vi "runBECBasic.vi"() -> ()   [LabVIEW 2011, in "run.lvlib"]
doc: "Launch the applications that will control the experiment.\n\n1) Load Database, filesystem, file neologist.\n2) Start a clock for the DDS rf card.\n3) Launch Experiment Runner front viewer\n4) Launch Hardware Controller in the backend."
uses:
  run.lvlib
  Viewers/Editors/ExperimentRunner/ExperimentRunner.lvclass
  HWController/HWController.lvclass
  HWController/BECHWCBasic/BECHWCBasic.lvclass
  HWController/HWControllerEvents/HWControllerEvents.lvclass
  Tools/DatabaseHelpers/DbConnection/DeviceDataBase/deviceDataBase.lvclass
  HWController/HardwareConfiguration/HWConfiguration.lvclass
  Viewers/Editors/ExperimentRunner/RunExperiment/ExperimentControl.lvclass
  Viewers/Editors/ExperimentRunner/Events/ExperimentControlEvents.lvclass
  HWController/AtomChipHWC/AtomChipHWC.lvclass
  Tools/Filing/FileSystem/FileSystem.lvclass
  Tools/Filing/FileNeologist/FileNeologist.lvclass
  Tools/Filing.lvlib
  Tools/DatabaseHelpers.lvlib
  Events/Event.lvclass
  Viewers/ExperimentControl.lvlib
panel:
  in  "Experiment":enum16{"BEC1", "AtomChip"}(ring)=enum."AtomChip"
  in  "Camera on?":bool
  in  "Hardware On?":bool=TRUE
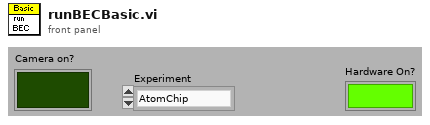
[diagram p1: front panel]
types:
  T1 = enum32{"Invalid", "Standard", "Closed", "Hidden", "Minimized", "Maximized"}
  T2 = enum32{"Bad", "Idle", "Run top level", "Running"}
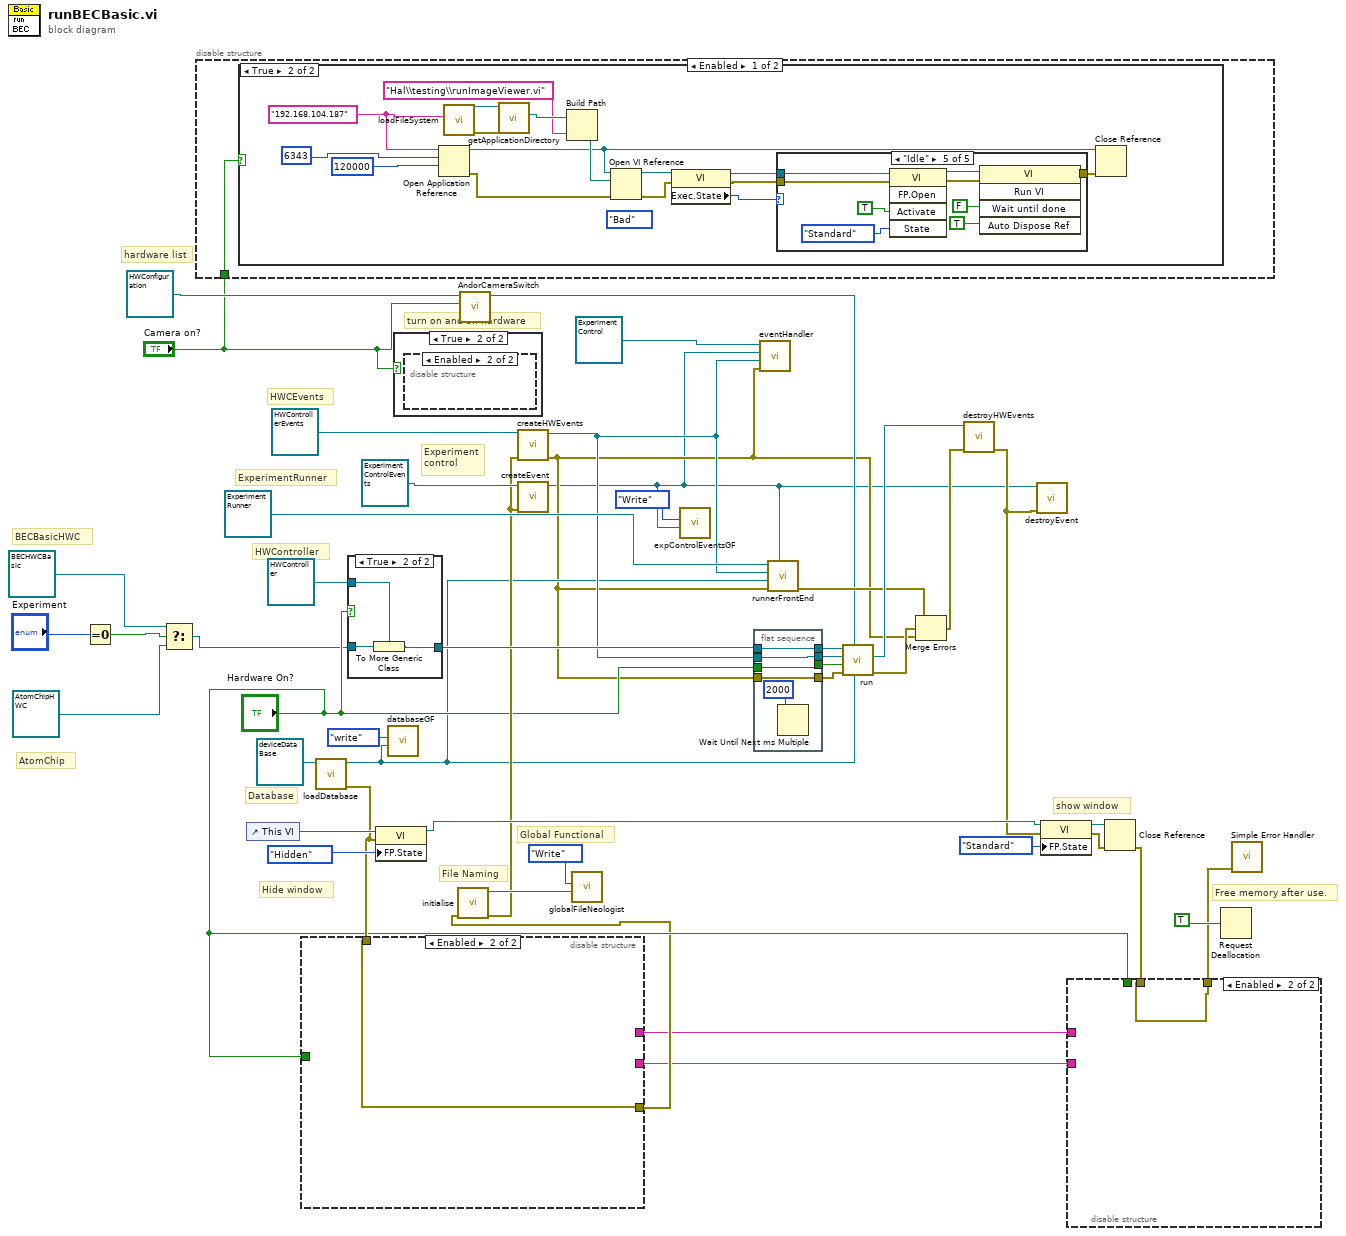
[diagram p0: block diagram]
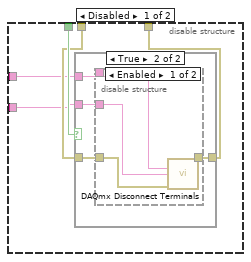
[diagram p8: hidden frame]
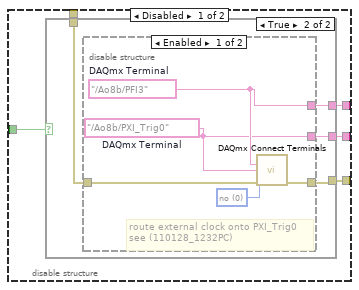
[diagram p11: hidden frame]
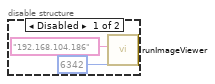
[diagram p15: hidden frame]
diagram:
  # "turn on and off hardware"
  # "AtomChip"
  # "Experiment\ncontrol"
  # "hardware list"
  # "Free memory after use."
  # "BECBasicHWC"
  # "Hide window"
  # "show window"
  # "Database"
  # "File Naming"
  # "Global Functional"
  # "HWController"
  # "ExperimentRunner"
  # "HWCEvents"
  n1 = Equal To 0?(x="Experiment") -> (x = 0?=w7:bool)
  n2 = Select(t=refnum<class "BECHWCBasic.lvclass"> refnum ("Hardware:HWControllers.lvlib:BECHWCBasic.lvclass"), s=w7, f=refnum<class "AtomChipHWC.lvclass"> refnum ("Hardware:HWControllers.lvlib:AtomChipHWC.lvclass")) -> (s? t:f=w4:refnum<class "HWController.lvclass">)
  n3 = disable-structure shown="Enabled" {
    disable-tunnel: "Camera on?" -> [w48 _]
    frame Enabled {
      n4 = case shown="True" w48 {
        frame False {
        }
        frame True {
          (unwired) T2."Bad" ("Execution:State")
          w55 = "192.168.104.187" ("remote address")
          n5 = Open Application Reference(9:120000 ("timeout ms (60000)"), 10:6343, 11:w55) -> (0:w64:errorcluster, 3:w58:refnum<vi>)  [unwired: 1 in]
          n6 = call "loadFileSystem.vi"("computer name"=w55) -> ("error out"=w62:errorcluster, "FileSystem out"=w63:refnum<class "FileSystem.lvclass">)  [unwired: 9 in]
          n7 = call-dynamic "getApplicationDirectory.vi"("error in (no error)"=w62, "FileSystem.lvclass in"=w63) -> ("ApplicationDirectory"=w61:path)  [unwired: 7 in, 2 out]
          n8 = Build Path(base path=w61, name or relative path="Hal\\testing\\runImageViewer.vi") -> (appended path=w59:path)
          n9 = Open VI Reference(application reference (local)=w58, vi path=w59, error in (no error)=w64) -> (vi reference=w53:refnum<vi>, error out=w52:errorcluster)  [unwired: 3 in]
          n10 = property class="VI"(reference=w53, error in=w52) -> (reference out=w50:refnum<vi>, error out=w51:errorcluster, "Exec.State"=w49:T2)
          n11 = case shown="\"Idle\"" w49 {
            tunnel: [w65 w66 w67 w68 w75] -> w57
            tunnel: w51 -> [w65 w66 w67 w68 w70]
            tunnel: w50 -> [_ _ _ _ w69]
            frame "Bad" {
            }
            frame Default {
            }
            frame "Running" {
            }
            frame "Run top level" {
            }
            frame "Idle" {
              n12 = invoke class="VI" method="FP.Open"(reference=w69, error in=w70, "Activate"=TRUE ("Activate?"), "State"=T1."Standard") -> (reference out=w71:refnum<vi>, error out=w72:errorcluster)  [unwired: 1 in, 3 out]
              n13 = invoke class="VI" method="Run VI"(reference=w71, error in=w72, "Wait until done"=FALSE, "Auto Dispose Ref"=TRUE ("Auto Dispose Reference")) -> (error out=w75:errorcluster)  [unwired: 1 in, 4 out]
            }
          }
          n14 = Close Reference(reference=w58, error in (no error)=w57) -> ()  [unwired: 1 out]
        }
      }
    }
    frame Disabled {
    }
  }
  n15 = control-ref of="This VI"() -> (w35:refnum<vi>)
  n16 = call "loadDatabase.vi"("deviceDataBase in"=refnum<class "deviceDataBase.lvclass"> refnum ("Tools.lvlib:DatabaseHelpers.lvlib:deviceDataBase.lvclass")) -> ("error out"=w18:errorcluster, "deviceDataBase out"=w10:refnum<class "deviceDataBase.lvclass">)  [unwired: 8 in, 1 out]
  n17 = disable-structure shown="Enabled" {
    disable-tunnel: w18 -> [w82 w94]
    disable-tunnel: "Hardware On?" -> [w81 _]
    disable-tunnel: [w80 w94] -> w16
    disable-tunnel: [w79 _] -> w13
    disable-tunnel: [w78 _] -> w12
    frame Disabled {
      n18 = case shown="True" w81 {
        tunnel: w82 -> [w83 w87]
        tunnel: [w83 w86] -> w80
        tunnel: [_ w85] -> w79
        tunnel: [_ w84] -> w78
        frame False {
        }
        frame True {
          n19 = disable-structure shown="Enabled" {
            disable-tunnel: w87 -> [w91 w93]
            disable-tunnel: [w90 w93] -> w86
            disable-tunnel: [w89 _] -> w85
            disable-tunnel: [w88 _] -> w84
            frame Enabled {
              w92 = 0 items=["no", "yes"] ("invert polarity")
              w88 = tag "/Ao8b/PXI_Trig0"  # DAQmx Terminal
              w89 = tag "/Ao8b/PFI3"  # DAQmx Terminal
              # "route external clock onto PXI_Trig0\nsee (110128_1232PC)"
              n20 = call <vilib>:"DAQmx Connect Terminals.vi"("source terminal"=w89, "destination terminal"=w88, "invert polarity"=w92, "error in"=w91) -> ("error out"=w90:errorcluster)  [unwired: 11 in]
            }
            frame Disabled {
            }
          }
        }
      }
    }
    frame Enabled {
    }
  }
  n21 = case shown="True" "Hardware On?" {
    tunnel: w4 -> [_ w98]
    tunnel: refnum<class "HWController.lvclass"> refnum ("Hardware:HWControllers.lvlib:HWController.lvclass") -> [w95 w97]
    tunnel: [w95 w96] -> w38
    frame False {
    }
    frame True {
      n22 = To More Generic Class(target class=w97, reference=w98) -> (generic class reference=w96:refnum<class "HWController.lvclass">)
    }
  }
  n23 = property class="VI"(reference=w35, error in=w18, "FP.State"=T1."Hidden" ("Front Panel Window:State")) -> (reference out=w26:refnum<vi>)  [unwired: 1 out]
  n24 = call "databaseGF.vi"("deviceDataBase in"=w10, "Enum"=enum16{"write", "read"}."write") -> ()  [unwired: 9 in, 1 out]
  n25 = case shown="True" "Camera on?" {
    frame False {
    }
    frame True {
      n26 = disable-structure shown="Enabled" {
        frame Disabled {
          n27 = call "runImageViewer.vi"("remote port"=u16 6342, "remote address"="192.168.104.186") -> ()  [unwired: 10 in]
        }
        frame Enabled {
        }
      }
    }
  }
  n28 = call "initialise.vi"("error in (no error)"=w16) -> ("error out"=w21:errorcluster, "FileNeologist out"=w30:refnum<class "FileNeologist.lvclass">)  [unwired: 9 in]
  n29 = call "AndorCameraSwitch.vi"("Andor Camera"="Camera on?", "HWConfiguration in"=refnum<class "HWConfiguration.lvclass"> refnum ("HardwareList out")) -> ("HWConfiguration out"=w23:refnum<class "HWConfiguration.lvclass">)  [unwired: 8 in, 1 out]
  n30 = call-dynamic "createHWEvents.vi"("error in (no error)"=w21, "HWControllerEvents in"=refnum<class "HWControllerEvents.lvclass"> refnum ("Hardware:HWControllers.lvlib:HWControllerEvents.lvclass")) -> ("error out"=w9:errorcluster, "HWControllerEvents out"=w11:refnum<class "HWControllerEvents.lvclass">)  [unwired: 8 in]
  n31 = call "createEvent.vi"("error in (no error)"=w21, "Event in"=refnum<class "ExperimentControlEvents.lvclass"> refnum ("ExperimentControlEvents")) -> ("Event out"=w2:refnum<class "ExperimentControlEvents.lvclass">)  [unwired: 8 in, 1 out]
  n32 = call "globalFileNeologist.vi"("FileNeologist in"=w30, "Action"=enum16{"Write", "Read"}."Write") -> ()  [unwired: 9 in, 1 out]
  n33 = call "expControlEventsGF.vi"("ExperimentControlEvents"=w2, "Action"=enum16{"Write", "Read"}."Write") -> ()  [unwired: 9 in, 1 out]
  n34 = flat-sequence {
    tunnel: [w104] -> w40
    tunnel: [w105] -> w39
    tunnel: w38 -> [w105]
    tunnel: w11 -> [w104]
    tunnel: [w103] -> w37
    tunnel: "Hardware On?" -> [w103]
    tunnel: [w102] -> w36
    tunnel: w9 -> [w102]
    frame #0 {
      n35 = Wait Until Next ms Multiple(millisecond multiple=2000) -> ()  [unwired: 1 out]
    }
  }
  n36 = call "eventHandler.vi"("error in (no error)"=w9, ":HWControllerEvents"=w11, "ExperimentControlEvents"=w2, "ExperimentControl in"=refnum<class "ExperimentControl.lvclass"> refnum) -> ()  [unwired: 6 in, 2 out]
  n37 = call "runnerFrontEnd.vi"("ExperimentControlEvents"=w2, "error in (no error)"=w9, "deviceDataBase"=w10, "HWControllerEvents"=w11, "Views.lvlib:ExperimentControl.lvlib:ExperimentRunner in"=refnum<class "ExperimentRunner.lvclass"> refnum ("Views.lvlib:ExperimentControl.lvlib:ExperimentRunner.lvclass")) -> ("error out"=w44:errorcluster)  [unwired: 5 in, 1 out]
  n38 = call "run.vi"("deviceDatabase"=w10, "HardwareList out"=w23, "error in (no error)"=w36, "debuggingFlag"=w37, "HWControllerEvents"=w40, "HWController in"=w39) -> ("error out"=w43:errorcluster, "HWControllerEvents out"=w45:refnum<class "HWControllerEvents.lvclass">)  [unwired: 3 in, 1 out]
  n39 = Merge Errors(w44, w43, w9) -> (w42:errorcluster)
  n40 = call-dynamic "destroyHWEvents.vi"("error in (no error)"=w42, "HWControllerEvents in"=w45) -> ("error out"=w20:errorcluster)  [unwired: 8 in, 1 out]
  n41 = call "destroyEvent.vi"("error in (no error)"=w20, "Event in"=w2) -> ()  [unwired: 8 in, 2 out]
  n42 = property class="VI"(reference=w26, error in=w20, "FP.State"=T1."Standard" ("Front Panel Window:State")) -> (reference out=w31:refnum<vi>, error out=w32:errorcluster)
  n43 = Close Reference(reference=w31, error in (no error)=w32) -> (error out=w15:errorcluster)
  n44 = disable-structure shown="Enabled" {
    disable-tunnel: "Hardware On?" -> [w110 _]
    disable-tunnel: w15 -> [w109 w121]
    disable-tunnel: [w108 w121] -> w14
    disable-tunnel: w13 -> [w107 _]
    disable-tunnel: w12 -> [w106 _]
    frame Disabled {
      n45 = case shown="True" w110 {
        tunnel: w109 -> [w111 w115]
        tunnel: [w111 w114] -> w108
        tunnel: w107 -> [_ w113]
        tunnel: w106 -> [_ w112]
        frame False {
        }
        frame True {
          n46 = disable-structure shown="Enabled" {
            disable-tunnel: w115 -> [w119 w120]
            disable-tunnel: [w118 w120] -> w114
            disable-tunnel: w113 -> [w117 _]
            disable-tunnel: w112 -> [w116 _]
            frame Enabled {
              n47 = call <vilib>:"DAQmx Disconnect Terminals.vi"("source terminal"=w117, "destination terminal"=w116, "error in"=w119) -> ("error out"=w118:errorcluster)  [unwired: 12 in]
            }
            frame Disabled {
            }
          }
        }
      }
    }
    frame Enabled {
    }
  }
  n48 = Request Deallocation(TRUE) -> ()
  n49 = call <vilib>:"Simple Error Handler.vi"("error in (no error)"=w14) -> ()  [unwired: 4 in, 5 out]
